vi "Read CCDCamera.lvclass.vi"(8 "error in (no error)":errorcluster, 11 "Image Constructor in":refnum<class "Simulated_Image_Constructor.lvclass">) -> (0 "error out":errorcluster, 2 "Simulated_CCD_Camera.lvclass":refnum<class "Simulated_CCD_Camera.lvclass">, 3 "Image Constructor out":refnum<class "Simulated_Image_Constructor.lvclass">)   [LabVIEW 2018, in "Simulated_Image_Constructor.lvclass"]
uses:
  Simulated_Image_Constructor.lvclass
  Simulated_CCD_Camera/Simulated_CCD_Camera.lvclass
  Simulated_Image_Constructor.lvclass/Simulated_Image_Constructor.ctl
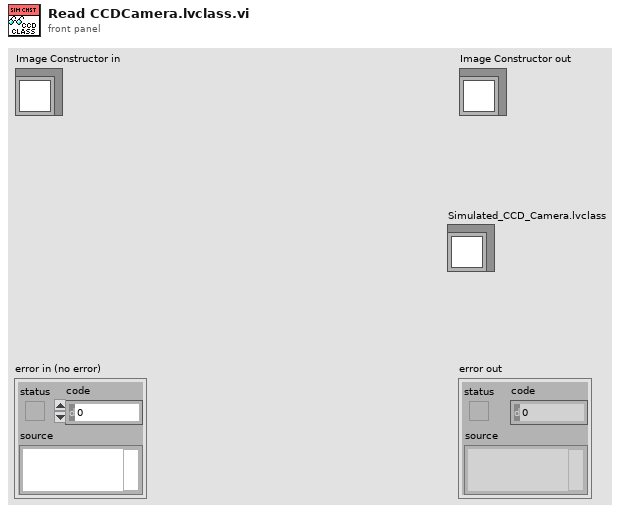
[diagram p1: front panel]
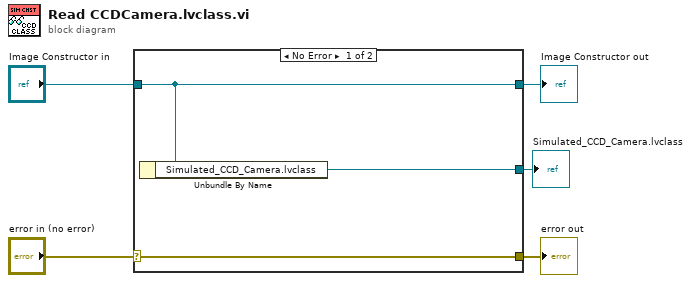
[diagram p0: block diagram]
diagram:
  n1 = case shown="No Error" "error in (no error)" {
    selector: "error in (no error)" -> [w8 w9]
    tunnel: [w8 w9] -> w4
    tunnel: [w7 w10] -> w2
    tunnel: "Image Constructor in" -> [w7 w10]
    tunnel: [w6 _] -> w1
    frame No Error {
      n2 = Unbundle By Name(w7) -> ("Simulated_CCD_Camera.lvclass"=w6:refnum<class "Simulated_CCD_Camera.lvclass">)
    }
    frame Error {
    }
  }
  "error out" <- w4
  "Image Constructor out" <- w2
  "Simulated_CCD_Camera.lvclass" <- w1
